vi "GyroBasedTurning.vi"(11 "Buttons":bool[](array[boolean])=[FALSE, FALSE, FALSE, FALSE, FALSE, FALSE, FALSE, FALSE, FALSE, FALSE]) -> (2 "RightMotors":dbl, 3 "LeftMotors":dbl)   [LabVIEW 2015]
uses:
  GlobalGyro.vi
  <vilib>/addons/control/pid/pid.llb/PID (DBL).vi
  <vilib>/addons/control/pid/NI_PID_pid.lvlib
panel:
  out "Angle":dbl
  in  "PID gains":T1={"proportional gain (Kc)"=5.0, "integral time (Ti, min)"=0.0, "derivative time (Td, min)"=0.0015} {"derivative time (Td, min)" format="%.5f"; "integral time (Ti, min)" format="%.3f"; "proportional gain (Kc)" format="%.3f"}
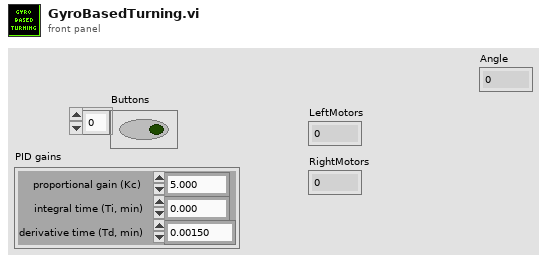
[diagram p1: front panel]
types:
  T1 = cluster{"proportional gain (Kc)":dbl, "integral time (Ti, min)":dbl, "derivative time (Td, min)":dbl}
  T2 = typedef "WPI_GyroDevRef.ctl" = cluster{"DevStatus":errorcluster, "Analog Channel":T3, "Offset":dbl, "Gain (VoltsPerDegree/Second)":dbl, "Gyro Type":enum16{"Analog", "XRS450"}, "Handle":i32, "SPI Bus":T4, "Device Found":bool, "Sample Rate":dbl, "Calibrate On Open":bool}
  T3 = typedef "FPGA_AIChannel.ctl" = enum8{"AI 0", "AI 1", "AI 2", "AI 3", "AI MXP 0", "AI MXP 1", "AI MXP 2", "AI MXP 3", "Invalid"}
  T4 = typedef "spi_bus.ctl" = enum16{"SPI On-Board, CS0", "SPI On-Board, CS1", "SPI On-Board, CS2", "SPI On-Board, CS3", "SPI MXP", "Invalid"}
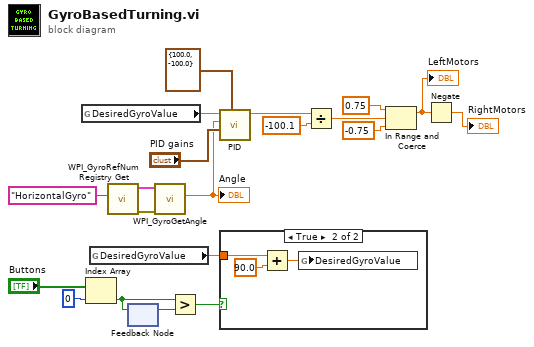
[diagram p0: block diagram]
diagram:
  n1 = global read "GlobalGyro.vi" "DesiredGyroValue"() -> (w1:dbl)
  n2 = Index Array(array="Buttons", index=0) -> (element=w4:bool)
  n3 = global read "GlobalGyro.vi" "DesiredGyroValue"() -> (w2:dbl)
  n4 = call <vilib>:"WPI_GyroRefNum Registry Get.vi"("refnum name"="HorizontalGyro") -> ("error out"=w18:errorcluster, "GyroDevRef"=w17:T2)  [unwired: 9 in]
  n5 = feedback-in #1(w4) -> ()
  n6 = feedback #1() -> (w5:bool)  [unwired: 1 in]
  n7 = call <vilib>:"WPI_GyroGetAngle.vi"("error in"=w18, "GyroDevRef"=w17) -> ("Angle"=w6:dbl)  [unwired: 5 in, 4 out]
  "Angle" <- w6
  n8 = Greater?(x=w4, y=w5) -> (0:w3:bool)
  n9 = call-poly <vilib>:"PID.vi"("output range"=cluster{"output high":dbl, "output low":dbl} {"output high"=100.0, "output low"=-100.0}, "PID gains"="PID gains", "process variable"=w6, "setpoint"=w1) -> ("output"=w13:dbl)  [unwired: 6 in, 1 out]
  n10 = case shown="True" w3 {
    tunnel: w2 -> [_ w23]
    frame False {
    }
    frame True {
      n11 = Add(x=w23, y=90.0) -> (x+y=w21:dbl)
      n12 = global write "GlobalGyro.vi" "DesiredGyroValue"(w21) -> ()
    }
  }
  n13 = Divide(x=w13, y=-100.1) -> (x/y=w11:dbl)
  n14 = In Range and Coerce(upper limit=0.75, x=w11, lower limit=-0.75) -> (coerced(x)=w8:dbl)  [unwired: 1 out]
  "LeftMotors" <- w8
  n15 = Negate(x=w8) -> (-x=→"RightMotors":dbl)
